vi "test_fft.vi"() -> ()   [LabVIEW 2009]
doc: "Copyright (c) 2010 Stepan A. Baranov (stepan@baranov.su)\nAll rights reserved.\nweb-site: www.OCTLab.org"
uses:
  <vilib>/Analysis/4window.llb/Hanning Window (DBL).vi
  <vilib>/Analysis/NI_AALPro.lvlib
  OCTLib_64.dll
panel:
  out "version":string
  out "name":string
  out "error out":errorcluster
  out "Im part":dbl[](array[numeric])
  out "Re part":dbl[](array[numeric])
  out "Phase A-scan":dbl[](array[numeric])
  out "Intensity A-scan":dbl[](array[numeric])
  out "Im":dbl[](array[numeric])
  out "Re":dbl[](array[numeric])
  out "phase":dbl[](array[numeric])
  out "intensity":dbl[](array[numeric])
  out "time for FFT":u32
  in  "RSM_STAT?":bool=TRUE
  in  "stop":bool
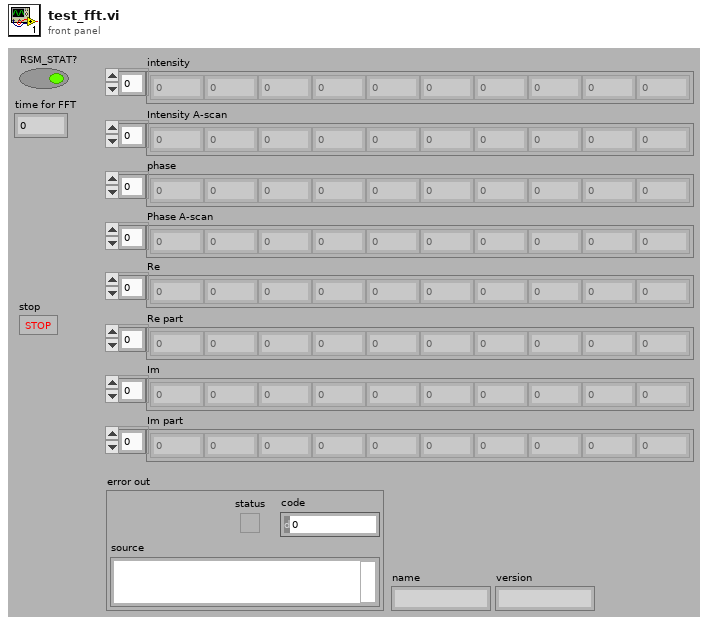
[diagram p1: front panel]
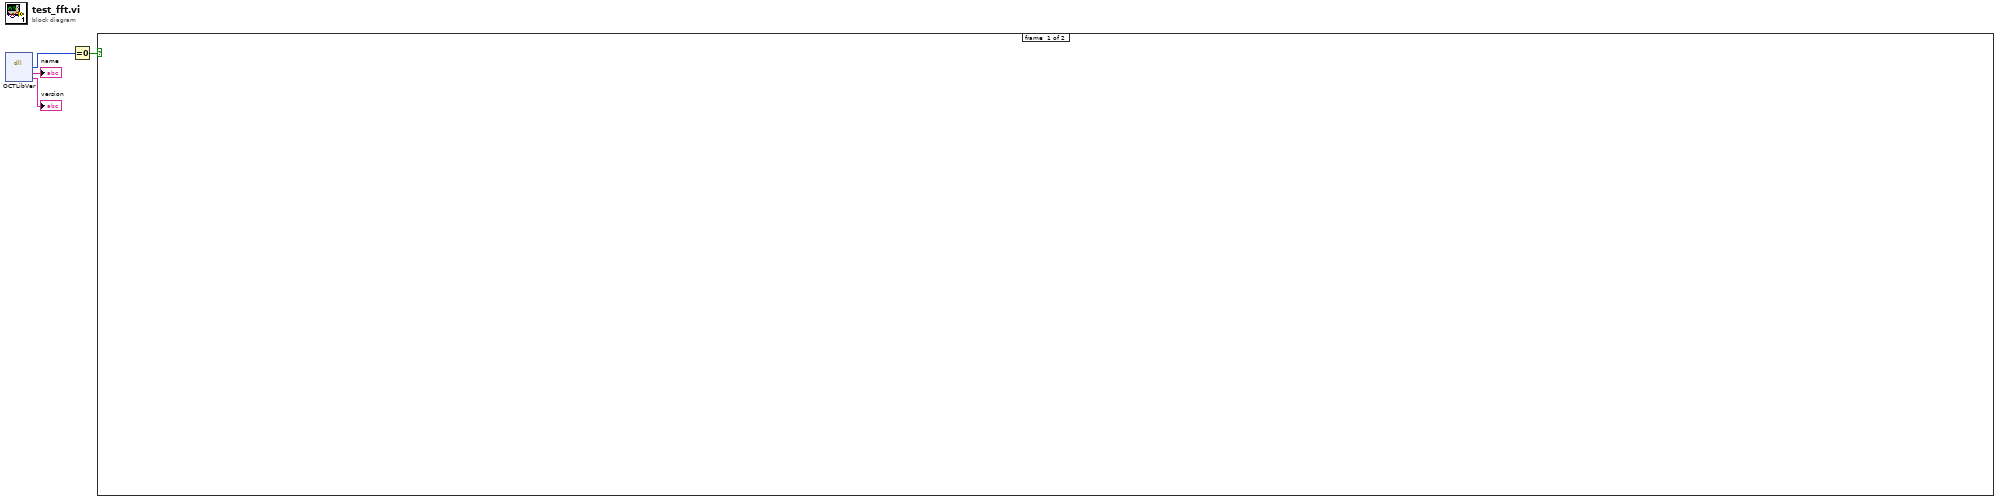
[diagram p0: block diagram]
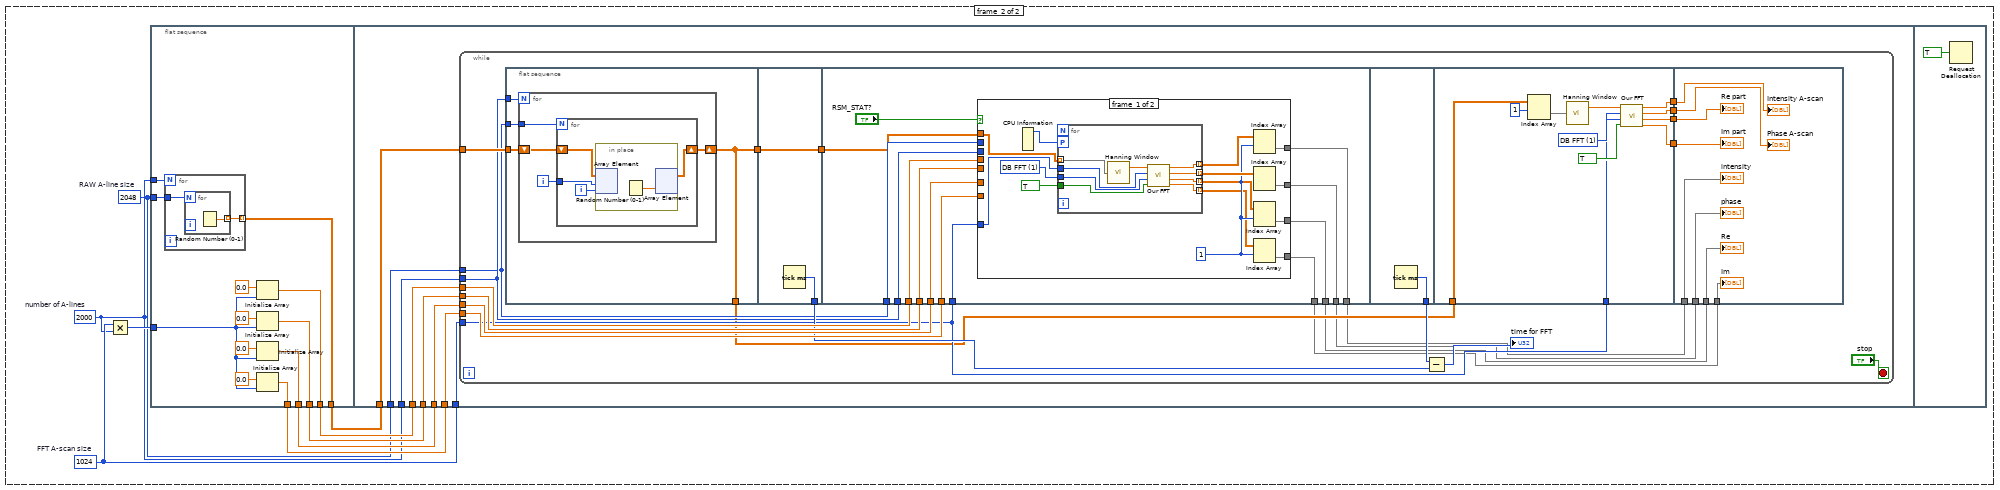
[diagram p2: hidden frame]
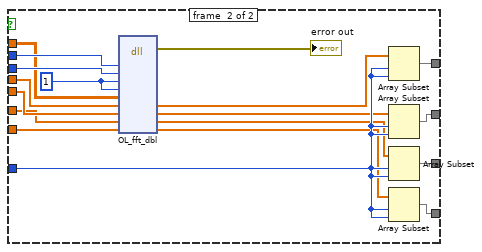
[diagram p3: hidden frame]
diagram:
  n1 = dll-call lib="OCTLib**.*" fn="OCTLibVer"() -> ("status"=w4:i8, "name"=→"name":string, "version"=→"version":string)  [unwired: 5 in, 2 out]
  n2 = Equal To 0?(x=w4) -> (x = 0?=w1:bool)
  n3 = case shown="True" w1 {
    frame #0 {
    }
    frame #1 {
      w7 = 1024  # FFT A-scan size
      w6 = 2000  # number of A-lines
      w5 = 2048  # RAW A-line size
      n4 = Multiply(x=w7, y=w6) -> (x*y=w13:i32)
      n5 = flat-sequence {
        tunnel: w5 -> [w25]
        tunnel: w6 -> [w24]
        tunnel: w13 -> [w19]
        tunnel: [w18] -> w12
        tunnel: [w17] -> w11
        tunnel: [w16] -> w10
        tunnel: [w15] -> w9
        tunnel: [w14] -> w8
        tunnel: w6 -> [w36]
        tunnel: w5 -> [w35]
        tunnel: w12 -> [w34]
        tunnel: w11 -> [w33]
        tunnel: w10 -> [w32]
        tunnel: w9 -> [w31]
        tunnel: w8 -> [w30]
        tunnel: w7 -> [w29]
        frame #0 {
          n6 = for {
            N: w24 -> [_]
            tunnel: [w27] -> w14 mode=indexing
            tunnel: w25 -> [w26]
            n7 = for {
              N: w26 -> [_]
              tunnel: [w28] -> w27 mode=indexing
              n8 = Random Number (0-1)() -> (number: 0 to 1=w28:dbl)
            }
          }
          n9 = Initialize Array(0.0 ("element"), w19) -> (w17:dbl[])
          n10 = Initialize Array(0.0 ("element"), w19) -> (w16:dbl[])
          n11 = Initialize Array(0.0 ("element"), w19) -> (w18:dbl[])
          n12 = Initialize Array(0.0 ("element"), w19) -> (w15:dbl[])
        }
        frame #1 {
          n13 = while {
            tunnel: w30 -> [w58]
            tunnel: w36 -> [w50]
            tunnel: w35 -> [w49]
            tunnel: w34 -> [w57]
            tunnel: w33 -> [w56]
            tunnel: w32 -> [w55]
            tunnel: w31 -> [w54]
            tunnel: w29 -> [w48]
            stop <- "stop" stop-if-true
            n14 = flat-sequence {
              tunnel: w58 -> [w63]
              tunnel: w50 -> [w62]
              tunnel: w49 -> [w61]
              tunnel: [w60] -> w47
              tunnel: [w60] -> w37
              tunnel: [w74] -> w53
              tunnel: [w73] -> w38
              tunnel: w37 -> [w73]
              tunnel: w57 -> [w86]
              tunnel: w56 -> [w85]
              tunnel: w55 -> [w84]
              tunnel: w54 -> [w83]
              tunnel: w49 -> [w82]
              tunnel: w50 -> [w81]
              tunnel: [w80] -> w42
              tunnel: [w79] -> w41
              tunnel: [w78] -> w40
              tunnel: [w77] -> w39
              tunnel: w48 -> [w76]
              tunnel: w38 -> [w75]
              tunnel: [w129] -> w51
              tunnel: w47 -> [w140]
              tunnel: w48 -> [w134]
              tunnel: [w133] -> w46
              tunnel: [w132] -> w45
              tunnel: [w131] -> w44
              tunnel: [w130] -> w43
              tunnel: w46 -> [w148]
              tunnel: w45 -> [w147]
              tunnel: w44 -> [w146]
              tunnel: w43 -> [w145]
              tunnel: w42 -> [w144]
              tunnel: w41 -> [w143]
              tunnel: w40 -> [w142]
              tunnel: w39 -> [w141]
              frame #0 {
                n15 = for {
                  N: w62 -> [_]
                  shift-right: [w65] -> w60
                  shift-left: w63 -> [w66]
                  tunnel: w61 -> [w67]
                  i -> [w64]
                  n16 = for {
                    N: w67 -> [_]
                    shift-right: [w68] -> w65
                    shift-left: w66 -> [w71]
                    tunnel: w64 -> [w70]
                    i -> [w69]
                    n17 = in-place {
                      n18 = in-place-array #1(w71, w70, w69) -> ()  [unwired: 1 out]
                      n19 = Random Number (0-1)() -> (number: 0 to 1=w72:dbl)
                      n20 = in-place-array #1(w72) -> (w68:dbl[][])  [unwired: 2 out]
                    }
                  }
                }
              }
              frame #1 {
                n21 = Tick Count (ms)() -> (millisecond timer value=w74:u32)
              }
              frame #2 {
                n22 = case shown="True" "RSM_STAT?" {
                  tunnel: w86 -> [_ w125]
                  tunnel: w85 -> [_ w128]
                  tunnel: w84 -> [_ w127]
                  tunnel: w83 -> [_ w126]
                  tunnel: w82 -> [_ w124]
                  tunnel: w81 -> [_ w123]
                  tunnel: w75 -> [w101 w121]
                  tunnel: [w98 w119] -> w80
                  tunnel: [w96 w116] -> w79
                  tunnel: [w95 w114] -> w78
                  tunnel: [w92 w112] -> w77
                  tunnel: w76 -> [w100 w120]
                  frame #0 {
                    w88 = 1 items=["LINEAR FFT", "DB FFT"] ("A-scan type")
                    w93 = 1 ("index (row)")
                    n23 = CPU Information() -> (4:w90:i32)  [unwired: 3 out]
                    n24 = for {
                      workers-P: w90 -> [_]
                      tunnel: [w109] -> w99 mode=indexing
                      tunnel: [w108] -> w97 mode=indexing
                      tunnel: [w107] -> w94 mode=indexing
                      tunnel: [w106] -> w91 mode=indexing
                      tunnel: w101 -> [w105] mode=indexing
                      tunnel: w100 -> [w104]
                      tunnel: TRUE ("need phase?") -> [w103]
                      tunnel: w88 -> [w102]
                      n25 = call-poly <vilib>:"Hanning Window.vi"("X"=w105) -> ("Windowed X"=w110:dbl[])  [unwired: 1 out]
                      n26 = call "Our FFT.vi"("need phase?"=w103, "A-scan type"=w102, "FFT A-scan size"=w104, "RAW A-line"=w110) -> ("Im part"=w106:dbl[], "Re part"=w107:dbl[], "Phase A-scan"=w108:dbl[], "Intensity A-scan"=w109:dbl[])
                    }
                    n27 = Index Array(array=w99, index (row)=w93) -> (element=w98:dbl[])  [unwired: 1 in]
                    n28 = Index Array(array=w97, index (row)=w93) -> (element=w96:dbl[])  [unwired: 1 in]
                    n29 = Index Array(array=w94, index (row)=w93) -> (element=w95:dbl[])  [unwired: 1 in]
                    n30 = Index Array(array=w91, index (row)=w93) -> (element=w92:dbl[])  [unwired: 1 in]
                  }
                  frame #1 {
                    w122 = i8 1 ("hanning_flag")
                    n31 = dll-call lib="OCTLib**.*" fn="OL_fft_dbl"("width"=w124, "height"=w123, "hanning_flag"=w122, "log10_flag"=w122, "input"=w121, "intensity"=w128, "phase"=w127, "Re"=w125, "Im"=w126) -> (error out=→"error out":errorcluster, "intensity"=w118:dbl[], "phase"=w117:dbl[], "Re"=w115:dbl[], "Im"=w113:dbl[])  [unwired: 9 in, 1 out]
                    n32 = Array Subset(array=w118, index=w120, length=w120) -> (w119:dbl[])
                    n33 = Array Subset(array=w117, index=w120, length=w120) -> (w116:dbl[])
                    n34 = Array Subset(array=w115, index=w120, length=w120) -> (w114:dbl[])
                    n35 = Array Subset(array=w113, index=w120, length=w120) -> (w112:dbl[])
                  }
                }
              }
              frame #3 {
                n36 = Tick Count (ms)() -> (millisecond timer value=w129:u32)
              }
              frame #4 {
                w137 = 1 items=["LINEAR FFT", "DB FFT"] ("A-scan type")
                n37 = Index Array(array=w140, index (row)=1) -> (element=w135:dbl[])  [unwired: 1 in]
                n38 = call-poly <vilib>:"Hanning Window.vi"("X"=w135) -> ("Windowed X"=w138:dbl[])  [unwired: 1 out]
                n39 = call "Our FFT.vi"("need phase?"=TRUE, "A-scan type"=w137, "FFT A-scan size"=w134, "RAW A-line"=w138) -> ("Im part"=w130:dbl[], "Re part"=w131:dbl[], "Phase A-scan"=w132:dbl[], "Intensity A-scan"=w133:dbl[])
              }
              frame #5 {
                "Intensity A-scan" <- w148
                "Phase A-scan" <- w147
                "Re part" <- w146
                "Im part" <- w145
                "intensity" <- w144
                "phase" <- w143
                "Re" <- w142
                "Im" <- w141
              }
            }
            n40 = Subtract(x=w51, y=w53) -> (x-y=→"time for FFT":u32)
          }
        }
        frame #2 {
          n41 = Request Deallocation(TRUE ("flag")) -> ()
        }
      }
    }
  }
